vi "fft_trial_v1.vi"() -> ()   [LabVIEW 2020]
uses:
  <vilib>/rvi/DataTransferAndStorage/Container/XNode/niFpgaContainer.xnode
  <vilib>/rvi/interface/RandomDataEmulation/nirviRandomDataFpgaReadWriteTemplate.vi
  <vilib>/rvi/FIFO/Fifo_Resource/niFpgaFifoEmulationRefIn.vi
  <vilib>/rvi/LocalResourceManager/LocalResourceManager.xnode
  <vilib>/rvi/eio/common/nirviEmuReportErrorAndStop.vi
  <vilib>/rvi/DataTransferAndStorage/Container/Common/niFpgaContainerGetUniqueNameForEmu.vi
  <vilib>/rvi/DataTransferAndStorage/Container/Common/niFpgaContainerSetEmuInfo.vi
  <resource>/lvanlys.dll
panel:
  out "FFT {X}":cdb[](array[numeric])
  out "error":i32
  in  "FFT size":i32=-1
  in  "shift?":bool
  out "Numeric 2":i32
  out "spectrum out":dbl[](array[numeric])
  out "df (Hz)":dbl
  in  "spectrum type":enum8{"Power (Vrms^2)", "Amplitude (Vrms)"}(ring)
  in  "imaginary FFT data":dbl[](array[numeric])
  in  "real FFT data":dbl[](array[numeric])
  in  "sample rate (S/s)":dbl format="%#_6p"
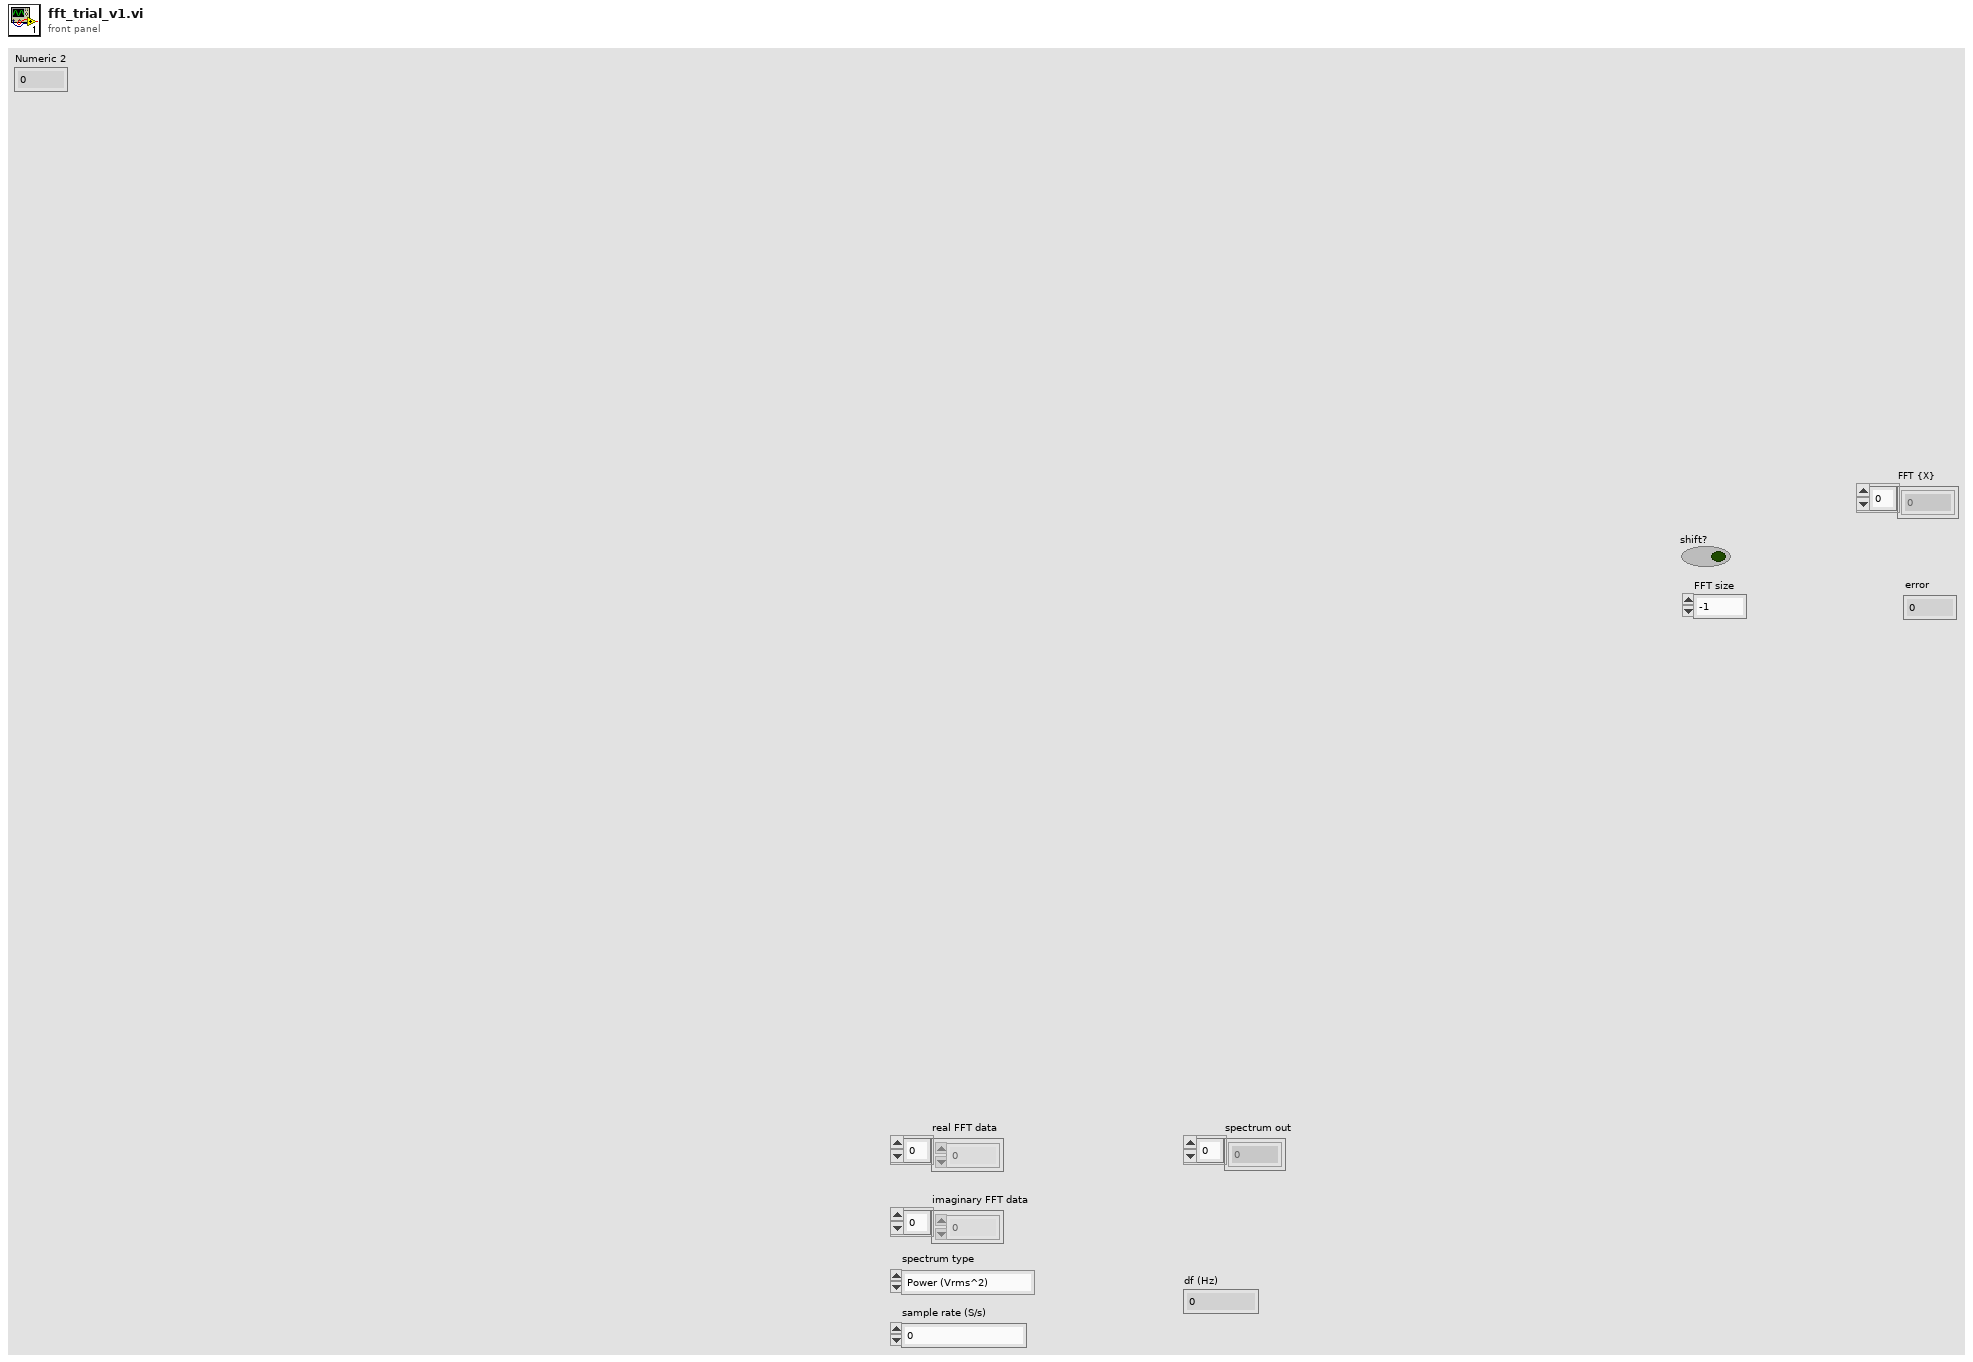
[diagram p1: front panel]
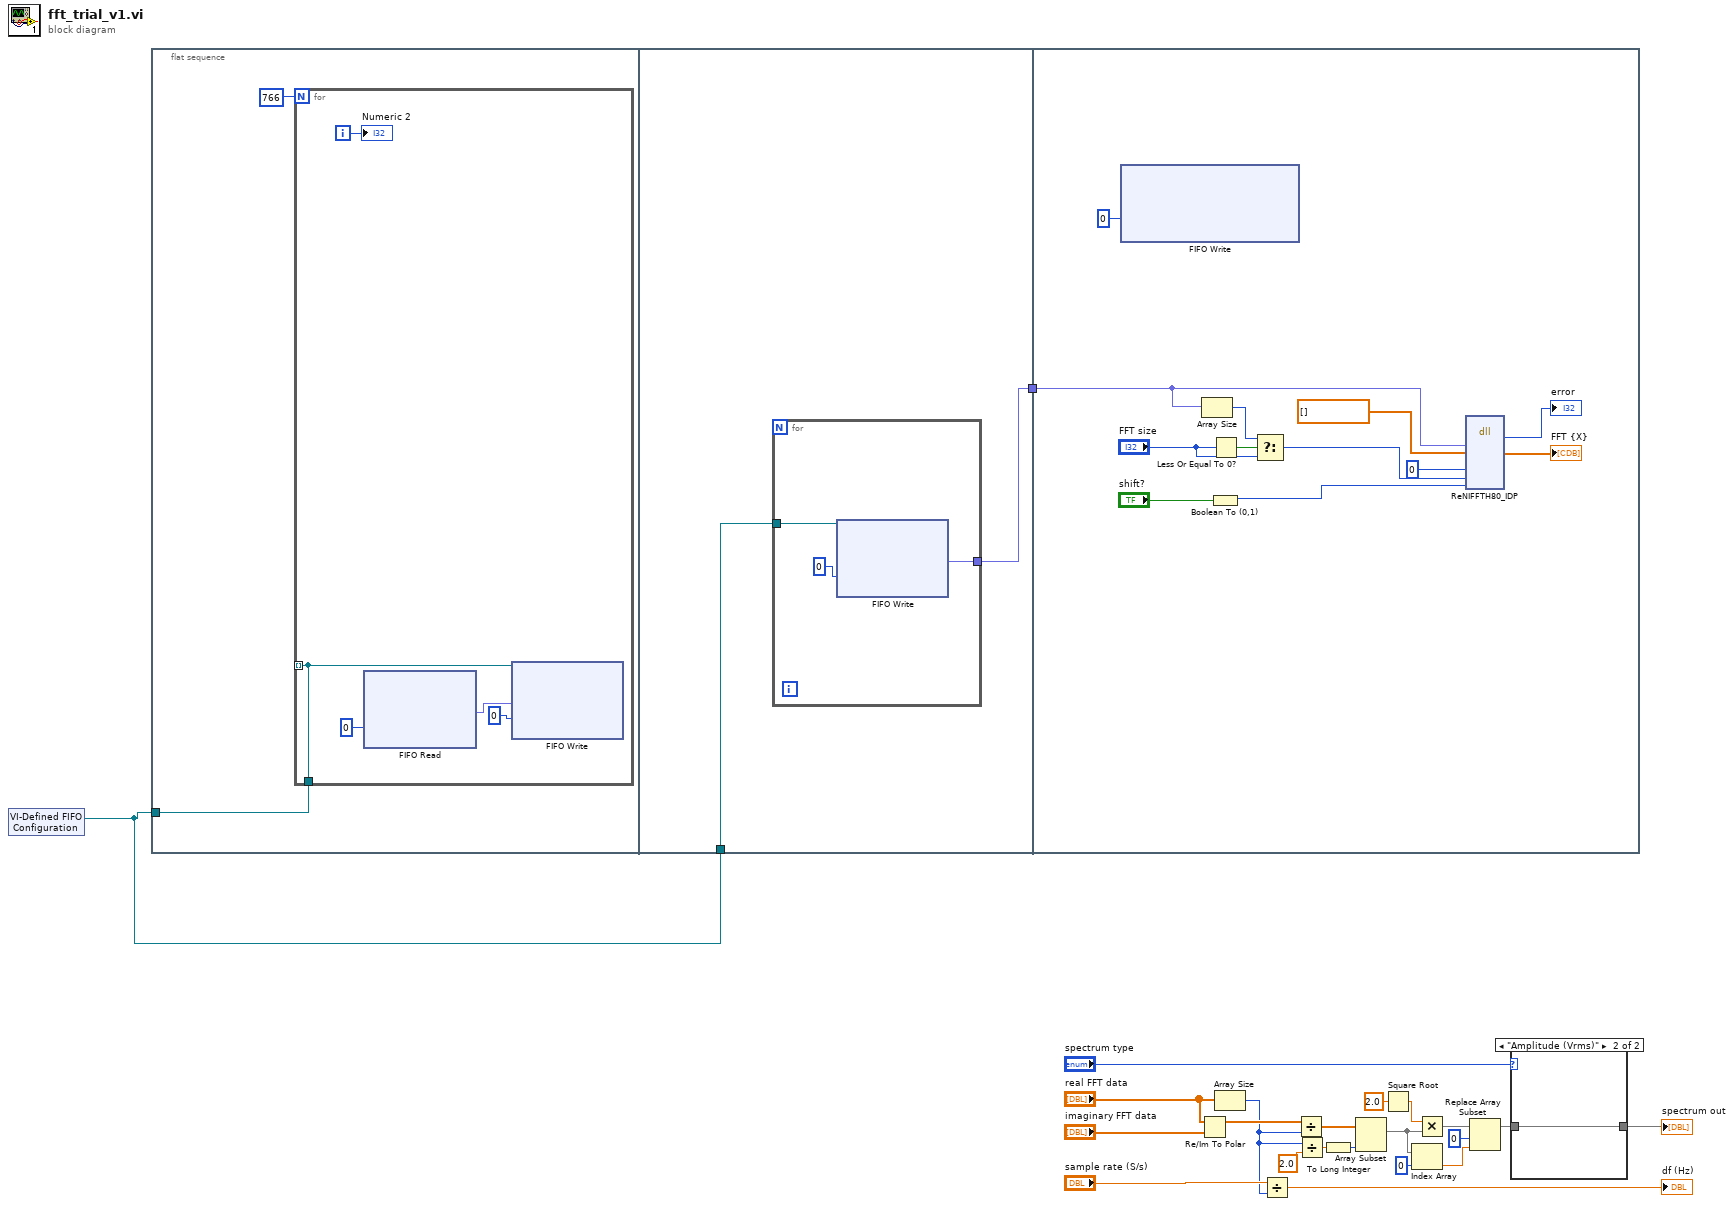
[diagram p0: block diagram]
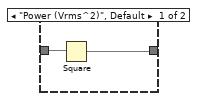
[diagram p2: hidden frame]
diagram:
  n1 = xnode "VI-Defined FIFO Configuration"() -> ("FIFO Out"=w2:refnum<k21>)
  n2 = flat-sequence {
    tunnel: w2 -> [w23]
    tunnel: w2 -> [w31]
    tunnel: [w30] -> w1
    tunnel: w1 -> [w35]
    frame #0 {
      n3 = for {
        N: 766 -> [_]
        tunnel: [w25] -> _ mode=indexing
        tunnel: w23 -> [w25]
        i -> [w26]
        n4 = xnode ("FIFO Read")("Timeout"=0) -> ("Element"=w27:fxp<+/-,24,7>)  [unwired: 1 in, 2 out]
        n5 = xnode ("FIFO Write")("Element"=w27, "Timeout"=0, "FIFO In"=w25) -> ()  [unwired: 2 out]
        "Numeric 2" <- w26
      }
    }
    frame #1 {
      n6 = for {
        tunnel: w31 -> [w34]
        tunnel: [w33] -> w30
        n7 = xnode ("FIFO Write")("Timeout"=0, "FIFO In"=w34) -> ("Element"=w33:fxp<+/-,24,7>)  [unwired: 2 out]
      }
    }
    frame #2 {
      n8 = xnode ("FIFO Write")("Timeout"=0) -> ()  [unwired: 2 in, 2 out]
      n9 = Array Size(array=w35) -> (size(s)=w44:i32)
      n10 = Boolean To (0,1)(Boolean="shift?") -> (0, 1=w40:i16)
      n11 = Less Or Equal To 0?(x="FFT size") -> (x <= 0?=w45:bool)
      n12 = Select(t=w44, s=w45, f="FFT size") -> (s? t:f=w43:i32)
      n13 = dll-call lib="C:/Program Files (x86)/National Instruments/LabVIEW 2020/resource/lvanlys.*" fn="ReNIFFTH80_IDP"("xH"=w35, "yH"=cdb[] [] ("FFT {X}"), "org"=0, "size"=w43, "shift"=w40) -> ("return type"=→"error":i32, "yH"=→"FFT {X}":cdb[])  [unwired: 9 in, 2 out]
    }
  }
  n14 = Re/Im To Polar(2:"imaginary FFT data", 3:"real FFT data") -> (1:w8:dbl[])  [unwired: 1 out]
  n15 = Array Size(array="real FFT data") -> (size(s)=w3:i32)
  n16 = Divide(x="sample rate (S/s)", y=w3) -> (x/y=→"df (Hz)":dbl)
  n17 = Divide(x=w8, y=w3) -> (x/y=w14:dbl[])
  n18 = Divide(x=w3, y=2.0) -> (x/y=w9:dbl)
  n19 = To Long Integer(number=w9) -> (32bit integer=w6:i32)
  n20 = Array Subset(array=w14, length=w6) -> (w11:dbl[])  [unwired: 1 in]
  n21 = Square Root(x=2.0) -> (sqrt(x)=w12:dbl)
  n22 = Index Array(array=w11, index=0) -> (element=w5:dbl)
  n23 = Multiply(x=w12, y=w11) -> (x*y=w13:dbl[])
  n24 = Replace Array Subset(array=w13, new element=w5, index=0) -> (w4:dbl[])
  n25 = case shown="\"Amplitude (Vrms)\"" "spectrum type" {
    tunnel: w4 -> [w48 w49]
    tunnel: [w47 w49] -> w17
    frame "Power (Vrms^2)", Default {
      n26 = Square(x=w48) -> (x^2=w47:dbl[])
    }
    frame "Amplitude (Vrms)" {
    }
  }
  "spectrum out" <- w17
